vi "FTW-Logger-Launch.vi"(5 "FTW Logger Configuration":string="{\n  \"Identity\": \"EventLog\",\n  \"InboxAddress\": \"inproc://*\",\n  \"PublisherAddress\": \"\",\n  \"LoggerAddress\": \"\",\n  \"DebugEnableInboxLogging\": false,\n  \"DebugEnableJobLogging\": false,\n  \"DebugShowPanel\": false,\n  \"ApplicationName\": \"Featherweight Application\",\n  \"LoggerName\": \"Log\",\n  \"LoggerDirectory\": \"[UserAppDir]\\\\Featherweight\\\\Logs\",\n  \"LoggerDiskThrashDelay\": 200\n}", 11 "error in":errorcluster) -> (4 "FTW Logger Connector":refnum<class "FTW-Logger.lvclass">, 6 "Logger Address":string, 15 "error out":errorcluster)   [LabVIEW 2013, in "FTW-Logger.lvclass"]
doc: "This method launches a Logger Process which is then referred to based on its LoggerID. Normally in a LabVIEW application, an object's methods would adhere to dataflow with the object wired to the method; however, the Logger Process object likely needs to be accessed by many different portions of your application, and for this reason, it is called by reference, where the LoggerID string refers to the logger.\n\nThis method should be called as one of the very first actions in your application to reasonably ensure the buffer of logged events does not overflow. Events that are logged prior to launching the Logger Process with this method are queued, and will be logged once this process begins."
uses:
  FTW-Logger.lvclass
  Connector/FTW-ActorConnector.lvclass
  Core/FTW-Logger-Core.lvclass
panel:
  in  "Boolean":bool
  # "Inputs"
  # "Outputs"
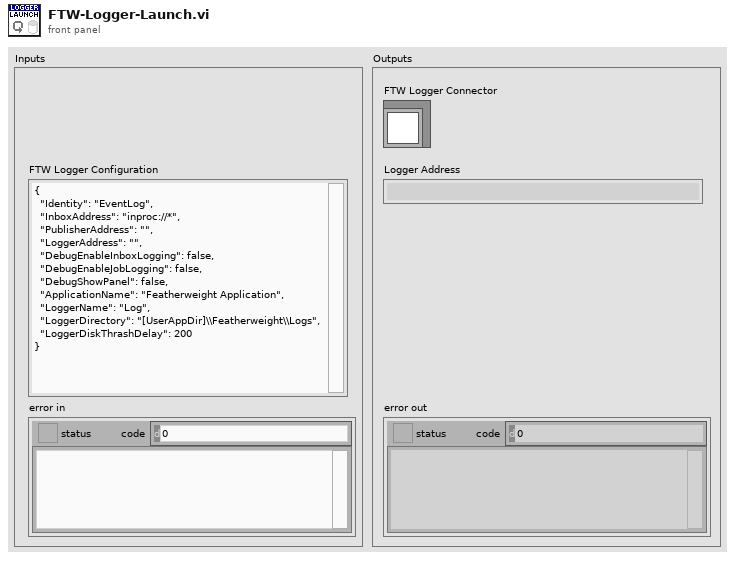
[diagram p1: front panel]
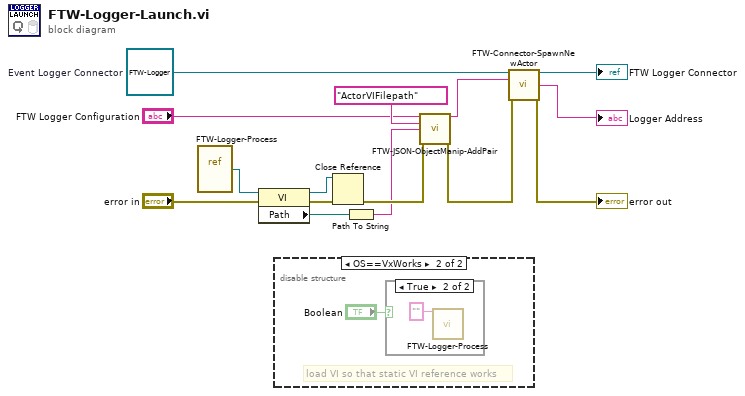
[diagram p0: block diagram]
diagram:
  w12 = refnum<class "FTW-Logger.lvclass"> refnum  # Event Logger Connector
  n1 = vi-ref "FTW-Logger-Process.vi"() -> (w10:refnum<vi>)
  n2 = property class="VI"(reference=w10, error in="error in") -> (reference out=w9:refnum<vi>, error out=w8:errorcluster, "Path"=w5:path)
  n3 = disable-structure shown="OS==VxWorks" {
    frame condition #0 (active) {
    }
    frame condition #1 {
      # "load VI so that static VI reference works"
      n4 = case shown="True" "Boolean" {
        frame False {
        }
        frame True {
          n5 = call "FTW-Logger-Process.vi"("FTW Logger Configuration"="" ("FTW Actor Instance Configuration")) -> ()  [unwired: 14 in, 1 out]
        }
      }
    }
  }
  n6 = Close Reference(reference=w9, error in (no error)=w8) -> (error out=w7:errorcluster)
  n7 = Path To String(path=w5) -> (string=w4:string)
  n8 = call "FTW-JSON-ObjectManip-AddPair.vi"("Input JSON Object"="FTW Logger Configuration", "Key"="ActorVIFilepath" ("JSON string to merge (\"\")"), "Value"=w4, "error in"=w7) -> ("Output JSON Object"=w1:string, "error out"=w6:errorcluster)  [unwired: 10 in]
  n9 = call "FTW-Connector-SpawnNewActor.vi"("FTW Actor Connector Type"=w12, "Configuration"=w1, "error in"=w6) -> ("FTW Actor Connector"=→"FTW Logger Connector":refnum<class "FTW-Logger.lvclass">, "Instance Inbox Address"=→"Logger Address":string, "error out"=→"error out":errorcluster)  [unwired: 9 in, 1 out]
